vi "test Add Find Remove RAF CD.vi"(8 "error in (no error)":errorcluster, 11 "TestCase in":refnum<class "Routing and Faulting Scripting Unit Tests.lvclass">) -> (0 "error out":errorcluster, 3 "TestCase out":refnum<class "Routing and Faulting Scripting Unit Tests.lvclass">)   [LabVIEW 2017, in "Routing and Faulting Scripting Unit Tests.lvclass"]
uses:
  Routing and Faulting Scripting Unit Tests.lvclass
  Routing and Faulting Scripting Unit Tests.lvclass/Routing and Faulting Scripting Unit Tests.ctl
  <vilib>/addons/_JKI Toolkits/VI Tester/TestCase.llb/TestCase.lvclass
  Routing and Faulting Scripting.lvlib
  C:/Program Files (x86)/National Instruments/LabVIEW 2017/vi.lib/addons/_JKI Toolkits/VI Tester/TestCase.llb/TestCase.lvclass
panel:
  in  "Save?":bool
  out "Output Filename":string
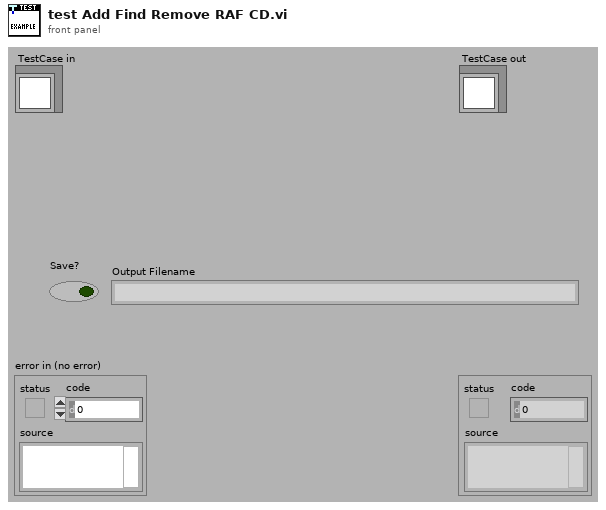
[diagram p1: front panel]
types:
  T1 = typedef "Custom Device API.lvlib/Custom Device Item Ref.ctl" = u64
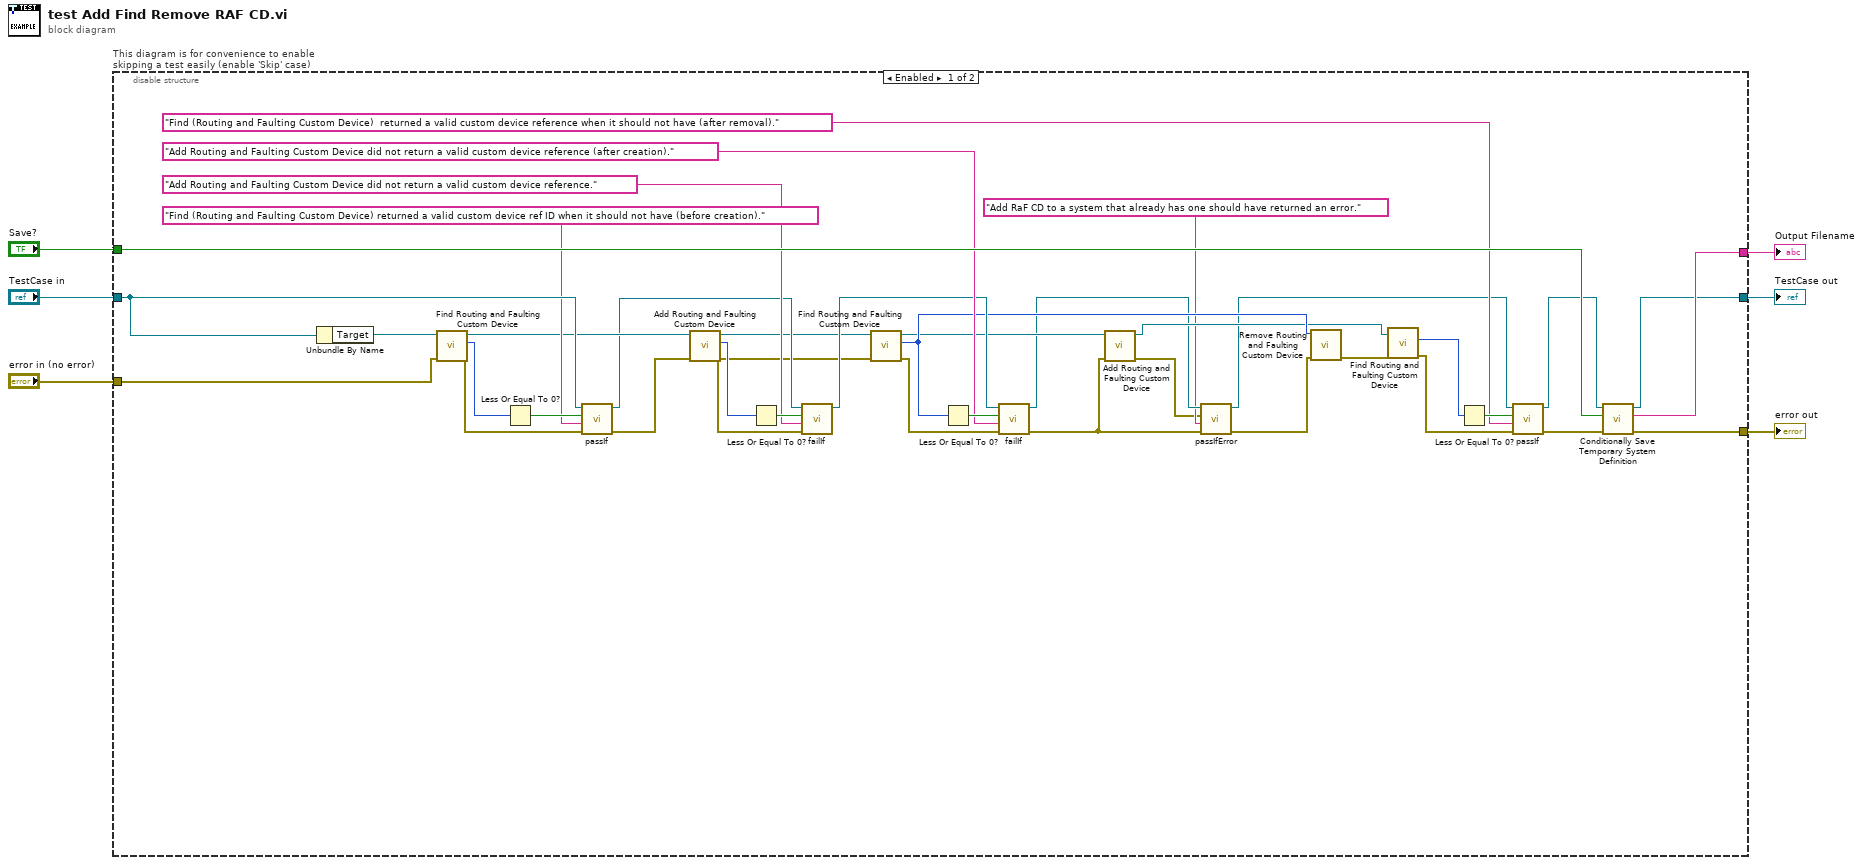
[diagram p0: block diagram]
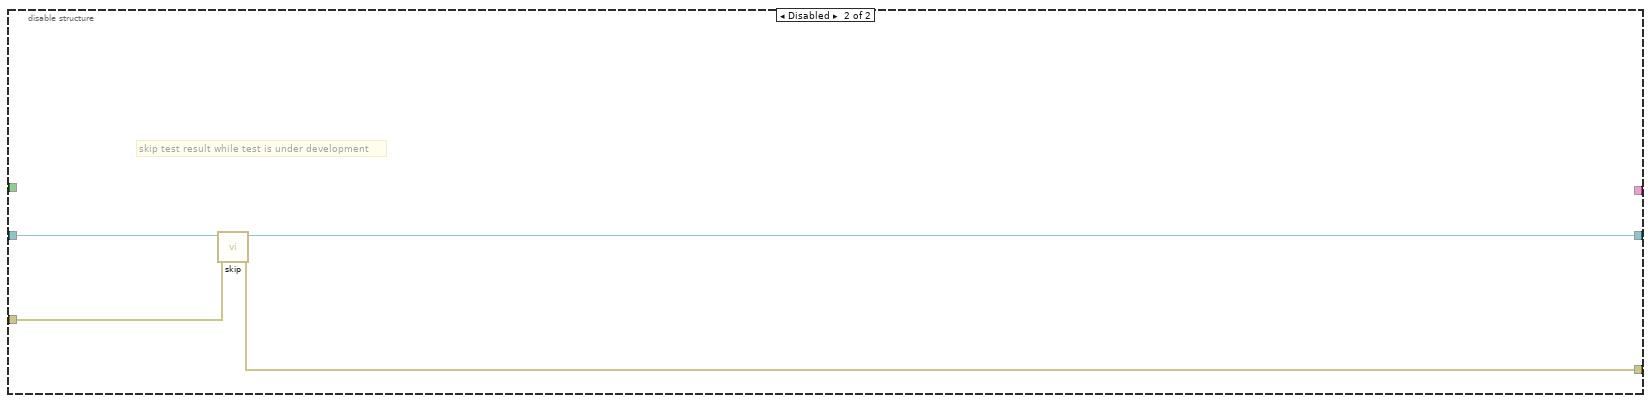
[diagram p2: hidden frame]
diagram:
  n1 = disable-structure "This diagram is for convenience to enable skipping a test easily (enable 'Skip' case)" shown="Enabled" {
    disable-tunnel: "TestCase in" -> [w39 w49]
    disable-tunnel: [w43 w47] -> w3
    disable-tunnel: [w44 w48] -> w5
    disable-tunnel: "error in (no error)" -> [w38 w46]
    disable-tunnel: [w45 _] -> w2
    disable-tunnel: "Save?" -> [w36 _]
    frame Enabled {
      n2 = Unbundle By Name(w39) -> ("Target"=w42:refnum<k24>)
      n3 = call "Find Routing and Faulting Custom Device.vi"("error in (no error)"=w38, "Target in"=w42) -> ("error out"=w37:errorcluster, "Routing and Faulting Custom Device Ref"=w41:T1, "Target out"=w34:refnum<k24>)  [unwired: 7 in]
      n4 = Less Or Equal To 0?(x=w41) -> (x <= 0?=w40:bool)
      n5 = call-dynamic "passIf.vi"("error in (no error)"=w37, "message (\"\")"="Find (Routing and Faulting Custom Device) returned a valid custom device ref ID when it should not have (before creation)." ("message (\"\")"), "pass"=w40, "TestCase in"=w39) -> ("error out"=w33:errorcluster, "TestCase out"=w13:refnum<class "Routing and Faulting Scripting Unit Tests.lvclass">)  [unwired: 6 in]
      n6 = call "Add Routing and Faulting Custom Device.vi"("error in (no error)"=w33, "Target in"=w34) -> ("error out"=w12:errorcluster, "Routing and Faulting Custom Device Ref"=w32:T1, "Target out"=w10:refnum<k24>)  [unwired: 7 in]
      n7 = Less Or Equal To 0?(x=w32) -> (x <= 0?=w31:bool)
      n8 = call-dynamic "failIf.vi"("error in (no error)"=w12, "message (\"\")"="Add Routing and Faulting Custom Device did not return a valid custom device reference." ("message (\"\")"), "fail"=w31, "TestCase in"=w13) -> ("TestCase out"=w27:refnum<class "Routing and Faulting Scripting Unit Tests.lvclass">)  [unwired: 6 in, 1 out]
      n9 = call "Find Routing and Faulting Custom Device.vi"("error in (no error)"=w12, "Target in"=w10) -> ("error out"=w11:errorcluster, "Routing and Faulting Custom Device Ref"=w26:T1, "Target out"=w18:refnum<k24>)  [unwired: 7 in]
      n10 = Less Or Equal To 0?(x=w26) -> (x <= 0?=w29:bool)
      n11 = call-dynamic "failIf.vi"("error in (no error)"=w11, "message (\"\")"="Add Routing and Faulting Custom Device did not return a valid custom device reference (after creation)." ("message (\"\")"), "fail"=w29, "TestCase in"=w27) -> ("error out"=w8:errorcluster, "TestCase out"=w16:refnum<class "Routing and Faulting Scripting Unit Tests.lvclass">)  [unwired: 6 in]
      n12 = call "Add Routing and Faulting Custom Device.vi"("error in (no error)"=w8, "Target in"=w18) -> ("error out"=w9:errorcluster, "Target out"=w17:refnum<k24>)  [unwired: 7 in, 1 out]
      n13 = call-dynamic "passIfError.vi"("error in (no error)"=w8, "task (\"\")"="Add RaF CD to a system that already has one should have returned an error." ("message (\"\")"), "error"=w9, "TestCase in"=w16) -> ("error out"=w7:errorcluster, "TestCase out"=w15:refnum<class "Routing and Faulting Scripting Unit Tests.lvclass">)  [unwired: 6 in]
      n14 = call "Remove Routing and Faulting Custom Device.vi"("error in (no error)"=w7, "Routing and Faulting Custom Device Ref"=w26) -> ("error out"=w25:errorcluster)  [unwired: 9 in]
      n15 = call "Find Routing and Faulting Custom Device.vi"("error in (no error)"=w25, "Target in"=w17) -> ("error out"=w23:errorcluster, "Routing and Faulting Custom Device Ref"=w21:T1)  [unwired: 7 in, 1 out]
      n16 = Less Or Equal To 0?(x=w21) -> (x <= 0?=w24:bool)
      n17 = call-dynamic "passIf.vi"("error in (no error)"=w23, "message (\"\")"="Find (Routing and Faulting Custom Device)  returned a valid custom device reference when it should not have (after removal)." ("message (\"\")"), "pass"=w24, "TestCase in"=w15) -> ("error out"=w19:errorcluster, "TestCase out"=w22:refnum<class "Routing and Faulting Scripting Unit Tests.lvclass">)  [unwired: 6 in]
      n18 = call "Conditionally Save Temporary System Definition.vi"("error in (no error)"=w19, "Save?"=w36, "Test Case"=w22) -> ("error out"=w44:errorcluster, "filename"=w45:string, "Test Case"=w43:refnum<class "Routing and Faulting Scripting Unit Tests.lvclass">)  [unwired: 6 in]
    }
    frame Disabled {
      # "skip test result while test is under development"
      n19 = call <vilib>:"skip.vi"("error in (no error)"=w46, "TestCase in"=w49) -> ("error out"=w48:errorcluster, "TestCase out"=w47:refnum<class "Routing and Faulting Scripting Unit Tests.lvclass">)  [unwired: 8 in]
    }
  }
  "error out" <- w5
  "TestCase out" <- w3
  "Output Filename" <- w2
